vi "Configure Peak Current Limits.vi"(0 "VISA resource name":refnum<visa-resource-name>, 5 "Current Peak Low Limit (0 A)":dbl min=0.0 max=152.0 format="%.3f", 7 "Current Peak High Limit (0 A)":dbl min=0.0 max=152.0 format="%.3f", 11 "error in (no error)":errorcluster) -> (4 "VISA resource name out":refnum<visa-resource-name>, 15 "error out":errorcluster)   [LabVIEW 2020, in "eec 6700.lvlib"]
doc: "Configures the current peak limits in the active step of the power source instrument.\n\n<B>Range</B> : 0.000~134.4 A\n\n0.0 ~16.8 A - 6705\n0.0 ~33.6 A - 6710\n0.0 ~67.2 A - 6720\n0.0 ~100.8 A - 6730\n0.0 ~134.4 A - 6740\n\nThe current peak Limit setting configures a peak current threshold level (High and Low Level). A test failure will occur when the high limit is reached or the low limit is not reached."
uses:
  <instrlib>/eec 6700/eec 6700.lvlib
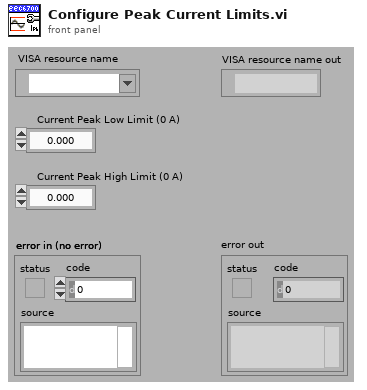
[diagram p1: front panel]
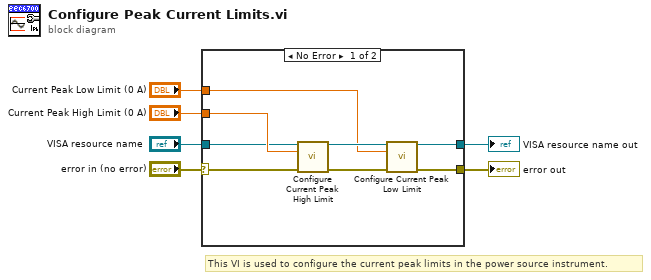
[diagram p0: block diagram]
diagram:
  # "This VI is used to configure the current peak limits in the power source instrument."
  n1 = case shown="No Error" "error in (no error)" {
    selector: "error in (no error)" -> [w7 w16]
    tunnel: [w13 w16] -> w6
    tunnel: [w12 w15] -> w5
    tunnel: "VISA resource name" -> [w8 w15]
    tunnel: "Current Peak High Limit (0 A)" -> [w10 _]
    tunnel: "Current Peak Low Limit (0 A)" -> [w9 _]
    frame No Error {
      n2 = call <instrlib>:"Configure Current Peak High Limit.vi"("VISA resource name"=w8, "Current Peak High Limit (0 A)"=w10, "error in (no error)"=w7) -> ("VISA resource name out"=w11:refnum<visa-resource-name>, "error out"=w14:errorcluster)  [unwired: 11 in]
      n3 = call <instrlib>:"Configure Current Peak Low Limit.vi"("VISA resource name"=w11, "Current Peak Low Limit (0 A)"=w9, "Error In"=w14) -> ("VISA resource name out"=w12:refnum<visa-resource-name>, "error out"=w13:errorcluster)  [unwired: 11 in]
    }
    frame Error {
    }
  }
  "error out" <- w6
  "VISA resource name out" <- w5
